vi "CRYChange Name by Calibratioin.vi"(9 "Calibration In":string, 10 "Hardware In":string, 11 "Changed Names":T2) -> ()   [LabVIEW 2013]
uses:
  CRYSystem/Typedef Control/CRYChanged Names Cluster.ctl
  CRYSystem/Typedef Control/CRYChanged Data Array Cluster.ctl
  CRYSystem/Typedef Control/CRYChanged Data Cluster.ctl
  CRYSystem/Typedef Control/CRYStimulus Type.ctl
  CRYCurveLibrary/Global/CRYCurve Library Global.vi
panel:
  in  "Ref Data Statistics":T1
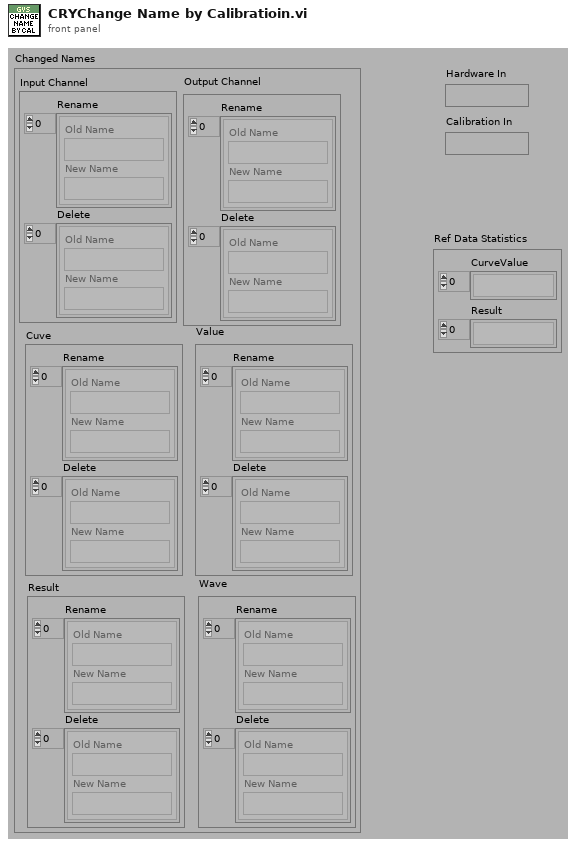
[diagram p1: front panel]
types:
  T1 = cluster{"CurveValue":string[], "Result":string[]}
  T2 = typedef "CRYChanged Names Cluster.ctl" = cluster{"Input Channel":T3, "Output Channel":T3, "Cuve":T3, "Value":T3, "Result":T3, "Wave":T3}
  T3 = typedef "CRYChanged Data Array Cluster.ctl" = cluster{"Rename":T4[], "Delete":T4[]}
  T4 = typedef "CRYChanged Data Cluster.ctl" = cluster{"Old Name":string, "New Name":string}
  T5 = typedef "CRYStep.ctl" = cluster{"No.VI":i32, "Category":string, "StepName":string, "Seq setup flattened":string, "Comment":string, "Steps config.":bool[], "Jump config":i32[], "Start":dbl, "Increment":dbl, "Name":string, "Unit":string, "Y data":u16, "Y prefix":string, "Y dB ref":dbl, "Y unit":string, "Repeat State Array":cluster{"Start":dbl, "Increment":dbl, "Count":i32, "Num":i32}[]}
  T6 = typedef "CRYStimulus Cluster.ctl" = cluster{"StimulusType":string, "UseMLValArray":u16[], "ML_axisArray":u16[], "MLValLevelNameArray":string[], "Level(U)Array":dbl[], "Start(Stop)FreqArray":dbl[], "Start(Stop)AmpArray":dbl[], "StepResolutionArray":u16[], "Unit_Array":u16[], "DegValArray":dbl[], "DegUnitArray":string[], "Steps1":i32, "Cycle/step1(#)":u32, "Time/step1(s)":dbl, "Transition1":dbl, "SweepRate2":dbl, "Freq3(Hz)":dbl, "Steps3(#)":dbl, "Cycles3(#)":u32, "StepSize3":dbl, "wave time":string, "RMS_Value4":dbl, "Peak_Value4":dbl, "WavePath4":string, "RMS_unit4":string, "Peak_unit4":string, "wave Info":string, "dc_ctrl5_1":u16, "dc_ctrl5_2":u16, "dc_polar5":u16, "Max.Current":u16, "Steps5(#)":u32, "Time/Step5":dbl, "Level5":dbl, "StepsSize5Val":dbl, "StepSize5Unit":string, "SweepType":u16, "Fixed/Ratio6":u16, "Transition6":dbl, "Steps6(#)":dbl, "Cycle/Steps6(#)":u32, "Time/Steps6(s)":dbl, "Freq6(Hz)":dbl, "Difference6(Hz)":dbl, "Ratio6":string, "NoiseType7":u16, "Duration7(s)":dbl, "MinFreq7(Hz)":dbl, "MaxFreq7(Hz)":dbl, "MinFreq8(Hz)":dbl, "MaxFreq8(Hz)":dbl, "FreqRounding8":bool, "Duration8(s)":dbl, "Tones8":dbl, "RoundingVal8":dbl, "ApplyEQ":bool, "Duration(s)":dbl, "CustomStimulusName ":string, "Flatten Element Array":string[], "sine waves":cluster{"freq":dbl, "ampl":dbl, "cycles":dbl}[], "Channel Out":i32, "RatioVal6":dbl, "TabCtrl6":enum32{"Master Tone", "Slave Tone"}, "Signal Type Name":string, "Help":string, "Channel Sel":u16, "V on DUT":bool, "Output Imp":dbl, "Nominal Imp":dbl}
  T7 = typedef "CRYfstepsw.ctl" = cluster{"Level(U)":dbl, "Start Freq(Hz)":dbl, "Stop Freq(Hz)":dbl, "ML val level name":string, "Use ML Val level?":bool, "ML axis":u8, "Steps (#)":i32, "Cycles/step(#)":u32, "Time/step (s)":dbl, "Step Resolution":u16, "unit":u16, "Start Freq Name":string, "Stop Freq Name":string, "Start Freq Axis":u8, "Stop Freq Axis":u8, "Start Freq Flag":string, "Stop Freq Flag":string, "Output Imp":dbl, "Nominal Imp":dbl, "V on DUT":bool}
  T8 = typedef "CRYflogsw.ctl" = cluster{"Level(U)":dbl, "Start Freq(Hz)":dbl, "Stop Freq(Hz)":dbl, "Sweep Rate(s/dec)":dbl, "Use ML Val level?":bool, "ML val level name":string, "ML axis":u8, "TSR params":cluster{"FSamp":dbl, "FStart":dbl, "FStop":dbl, "NOffset":dbl, "MStop":dbl, "MStart":dbl, "NHarm":dbl, "Tsamp":dbl, "Amplit":dbl}, "unit":u16, "Start Freq Name":string, "Stop Freq Name":string, "Start Freq Axis":u8, "Stop Freq Axis":u8, "Start Freq Flag":string, "Stop Freq Flag":string, "Output Imp":dbl, "Nominal Imp":dbl, "V on DUT":bool}
  T9 = typedef "CRYampsw.ctl" = cluster{"Freq(Hz)":dbl, "Steps (#)":i32, "Cycles(#)":u32, "Use ML Val freq?":bool, "ML val freq name":string, "ML axis":u8, "Start Ampl(U)":dbl, "Stop Ampl(U)":dbl, "unit":u16}
  T10 = typedef "CRYwavefile.ctl" = cluster{"Level(U)":dbl, "Wave Path":string, "ML axis":u8, "ML val level name":string, "Use ML Val level?":bool, "wave info":string, "wave time":string, "Peak value4":dbl, "RMS value4":dbl, "wave channel":u16, "unit":u16, "Output Imp":dbl, "Nominal Imp":dbl, "V on DUT":bool}
  T11 = typedef "CRYdcconn.ctl" = cluster{"dc ctrl":u16, "dcmax I":u16, "dc polar":u16, "dc ctrl":u16, "Steps (#)":i32, "Time/step (s)":dbl, "Start Ampl(U)":dbl, "Stop Ampl(U)":dbl, "Level(U)":dbl, "Step Size":dbl}
  T12 = typedef "CRYtwotone.ctl" = cluster{"Steps (#)":i32, "Tone Type":u8, "Freq2(Hz)":dbl, "Time/step (s)":dbl, "Cycles/step (#)":u32, "ML val level name":string, "Use ML Val level?":bool, "Level(U) 2":dbl, "Diff Freq(Hz)":dbl, "ML axis 2":u8, "Diff/Ratio":u8, "Level(U)":dbl, "Stop Freq(Hz)":dbl, "Ratio Val":dbl, "ML val level name 2":string, "Use ML Val level? 2":bool, "ML axis":u8, "Start Freq(Hz)":dbl, "Step Resolution":u16, "Ratio":u16, "TabCtrl6":enum32{"Master Tone", "Slave Tone"}, "unit 1":u16, "unit 2":u16, "Start Freq Name":string, "Stop Freq Name":string, "Start Freq Axis":u8, "Stop Freq Axis":u8, "Start Freq Flag":string, "Stop Freq Flag":string}
  T13 = typedef "CRYmltitone.ctl" = cluster{"Level(U)":dbl, "Min Freq(Hz)":dbl, "Max Freq(Hz)":dbl, "Duration(s)":dbl, "Freq Rounding":bool, "Rounding Val":dbl, "Profile":i32, "ML axis 2":u8, "ML val level name":string, "Use ML Val level?":bool, "ML axis":u8, "Step Resolution":u16, "unit":u16, "Start Freq Name":string, "Stop Freq Name":string, "Start Freq Axis":u8, "Stop Freq Axis":u8, "Start Freq Flag":string, "Stop Freq Flag":string, "Output Imp":dbl, "Nominal Imp":dbl, "V on DUT":bool}
  T14 = typedef "CRYnoise.ctl" = cluster{"Noise Type":u8, "Min Freq(Hz)":dbl, "Max Freq(Hz)":dbl, "Level(U)":dbl, "Duration(s)":dbl, "ML val level name":string, "Use ML Val level?":bool, "ML axis":u8, "unit":u16, "Start Freq Name":string, "Stop Freq Name":string, "Start Freq Axis":u8, "Stop Freq Axis":u8, "Start Freq Flag":string, "Stop Freq Flag":string, "Output Imp":dbl, "Nominal Imp":dbl, "V on DUT":bool}
  T15 = cluster{"fstepsw":T7, "flogsw":T8, "ampsw":T9, "wavefile":T10, "dcconn":T11, "twotone":T12, "mltitone":T13, "noise":T14, "sqwvsw":cluster{"Level(U)":dbl, "Duty Cycle":dbl, "ML val level name":string, "ML axis":u8, "Start Freq(Hz)":u32, "Stop Freq(Hz)":u32, "Use ML Val level?":bool, "Steps (#)":u32, "Cycles/step (#)":u32, "Time/step (s)":dbl, "Step Resolution":u16}, "tnbrst":cluster{"Level(U)":dbl, "ML val level name":string, "ML axis":u8, "Start Freq(Hz)":u32, "Use ML Val level?":bool, "Cycles/step (#)":u32, "Duration(s)":dbl}}
  T16 = cluster{"Data Type":string, "Version":u16, "Dimension":u8}
  T17 = typedef "CRYStimulus Type.ctl" = u16
  T18 = typedef "CRYAcquisition Cluster.ctl" = cluster{"Mode":u16, "Name":string, "use ch name":bool, "Record Time":dbl, "hide rec":bool, "hide play":bool, "rec delay":dbl, "rec pad":dbl, "dcc units":i8, "sine gen setting":string, "scope_fft setting":string, "voltmeter setting":string, "rta setting":string, "trig offset(sec)":dbl, "triggered  record":bool, "trig level":dbl, "trig unit":u8, "trig slop":bool, "trig timeout(sec)":dbl, "add record":bool, "EQ":bool, "record table":string[][], "play table":string[][], "trig channel":string, "Help":string}
  T19 = typedef "CRYAnalysis Cluster.ctl" = cluster{"Name":string, "Harmonics":dbl[], " Algorithm":u16, "delay":dbl, "THD(%)":bool, "Rub&Buzz":bool, "Imp":bool, "Imp Ref resistor":dbl, "Y data":u16, "Y prefix":string, "Y unit":string, "Y dB ref":dbl, "Custom Curve Names":string[], "har list items":string[], "Envelope":bool, "use custom unit":bool, "autodelay ch":dbl, "impulse":bool, " start ms":dbl, " stop ms":dbl, "Scaling":i32, "Default Overlap ":bool, "Advanced View":bool, "Loose Particle":bool, "Use default":bool, "Auto-Correlation(Stimulus)":bool, "Auto-Correlation(Response)":bool, "Deconvolved Response":bool, "Mic Current":bool, "M List Vaiues":u16, "Type":u16, "Delay Method":u16, "Apply Correction Out":bool, "Apply Correction In":bool, "Harmonics @ meas.frq":bool, "THD Normalized(%)":bool, "Total Distortion":bool, "THD+Noise(%)":bool, "Rub&Buzz Norm'd(%)":bool, "Standard Error":bool, "Confidence Limits":bool, "Total Diff":bool, "Total Noise":bool, "Total DFD(%)":bool, "Total IMD(%)":bool, "Total IM":bool, "Total DFD+Noise(%)":bool, "Use Channel Name":bool, "Waveform In":string, "Waveform Out":string, "Method":u16, "Spectral Scaling":u16, "Appliied Unit":u16, "Length Unit":u16, "Applied Units":u16, "Sens Item":u16, "Tab":i32, "Distance Unit":u16, "discard cycles":dbl, "Weigting":string, "Averaging Time":dbl, "Max duration":dbl, "Min duration":dbl, "Attack Threshold":dbl, "Hysteresis Up":dbl, "Fmin(Hz)":dbl, "Fmax(Hz)":dbl, "Freq.Resolution":dbl, "Over-samples Res.":dbl, "Win Resolution":dbl, "distance":dbl, "samples":dbl, "Overlap":dbl, "Record Length":dbl, "No.of FFTs":dbl, "Hz":dbl, "record delay":dbl, " Std Err":dbl, "Response":bool, "Coherent Power*":bool, "Stimulus":bool, "Measurement Confidence":bool, "Auto Spectrum(Response)*":bool, "Auto Spectrum(Stimulus)*":bool, "Cross Spectrum*":bool, "functions":bool, "Frequency Response":bool, "Non-Coherent Power*":bool, "Coherence (%)":bool, "Non-Coherence (%)":bool, "Signal-Noise Ratio (dB)":bool, "Non-Coherenct Distirtion*":bool, "Result Waveforms":bool, "Coupling":bool, "Averaging":u16, "Harmonics":i32, "Custom Curve Names":i32, "unLabel":string, "Custom Curve Names":string, "Unit":string, "Total IMD + Noise(%) ":bool, "ResponseMe":u16, "Intermod":dbl[], "Diff\n":dbl[], "Cross-Correlation":bool, "IM list items":string[], "Diff list items":string[], "TSR Window Type":string, "Help":string, "Custom Curve IDs":i32[], "Default Curve Names":string[], "Loose Particle waveform":bool, "Perceptual Rub&Buzz":bool, "Imp Auto Mode":u16, "Mic Auto Mode":u16, "Mic Ref resistor":dbl, "Curve Resolution":u16, "Curve Resolution Hz":dbl, "Polarity":bool}
  T20 = typedef "CRYWaveform Cluster.ctl" = cluster{"Waveform":cluster{"X0":dbl, "dX":dbl, "Y":sgl[]}, "X data":u16, "Y data":u16, "Y axis":u16, "X unit":string, "Y unit":string, "Y dB ref":dbl, "display Y":bool, "display X":bool, "Overload?":bool, "Test Info":string, "Step No.":i32, "Name":string, "protected":bool, "Sqc history":string[], "Signal Channel ID":i32, "Plot Settings":cluster{"Color":u32, "Interpolation":u8, "Point Style":u8, "Line Style":u8, "Point Color":u32, "Line Width":u8, "Bar Plot Style":u8, "Fill To":i16}, "AutoProtect":bool}
  T21 = typedef "CRYStimulus Test Infor Cluster.ctl" = cluster{"Stimulus Type":string, "Signal Type":string, "In/Out":bool, "FAPS":cluster{"freq":dbl, "ampl":dbl, "cycles":dbl, "samples":i32}[], "Sampling Rate":dbl, "Samples":i32, "Analysis Param":string, "Resolution":u16, "Steps":u32, "Analysis Value":dbl[], "Diff Freq":dbl, "FStart":dbl, "FStop":dbl, "Calibration Param":string, "Anti Alias":dbl, "Level Out1":dbl, "Level Out2":dbl, "EQ":bool}
  T22 = cluster{"Custom Curve Names":string, "Custom Curve IDs":i32, "Default Curve Names":string}[]
  T23 = typedef "CRYPost Processing Cluster.ctl" = cluster{"Name":string, "Op Type":u16, "Curve A":string, "Curve B":string, "Axis Mode":u16, "Work Mode":u16, "Width":u16, "Weighting win":u16, "Search Mode":u16, "Freq Mode":u16, "New Sampling Rate":dbl, "Use Default Name":bool, "x":bool, "y":bool, "z":bool, "All points":bool, "A_single val axis":u16, "B_single val axis":u16, "Use Default Value":bool, "Result Name":string, "Smoothing Width":i32, "Window":u16, "Para_dB":sgl, "Para_%":sgl, "Exponent":sgl, "Hz":dbl, "Direct Weighting":bool, "Auto Inc":bool, "Inc(deg)":i32, "Total Rotation":i32, "Ref Freq Mode":u16, "Ref Waveform":string, "Sampling Rate":dbl, "Weighting Curve":string, "Ref Freq":dbl, "Curve Group":string[], "Search Items":string[], "Custom unit info":cluster{"use custom":bool, "lin/log":u16, "unit":string, "dB ref":dbl, "common dB":u16}, "Unit":string, "Type A":enum16{"Curves", "Values", "Results", "WFM"}, "Type B":enum16{"Curves", "Values", "Results", "WFM"}, "Unary Operator":u16, "Binary Operator":u16, "Statistical Operator":u16, "Constant ":dbl, "New Resolution":u16, "user equation cluster":T24, "Help":string, "Tab Value":enum32{"Setting", "Help"}, "Zwciker_X-axis":u16, "Zwicker_spectrum":bool, "Freq Sampling Mode":u16, "Freq Sampling Rate":dbl, "Smoothing":bool, "Work in Statics":u16, "Result Data":string[]}
  T24 = typedef "CRYUser Equation Cluster.ctl" = cluster{"Custom unit input array":cluster{"use custom":bool, "lin/log":u16, "unit":string, "dB ref":dbl, "common dB":u16}[], "Custom unit results array ":cluster{"use custom":bool, "lin/log":u16, "unit":string, "dB ref":dbl, "common dB":u16}[], "Desired Result Variables":string[], "Desired Result Names":string[], "Input Curve Names":string[], "Input Curve Variables":string[], "equation":string, "Input axis":u16[], "Results axis":u16[], "# input curves":i32, "# Desired result curves ":i32, "Input Values":string[], "Result Values":string[]}
  T25 = typedef "CRYLimits.ctl" = cluster{"Name":string, "Tolerance":u16, "X Axis":u16, "Limits":u16, "Upper Limit":cluster{dbl, dbl}[], "Align Ref":cluster{dbl, dbl}, "Lower Limit":cluster{dbl, dbl}[], "Y data":u16, "Y unit":string, "Y dB ref":dbl, "Curve Names":string[], "Y-Resolution":u8, "Type":u16, "x float":bool, "X min-max-step":cluster{"Limit X Offset Min":dbl, "Limit X Offset Max":dbl, "Limit X Offset Step Size":dbl}, "magn/phase":u16, "Upper Limit Type":u16, "Lower Limit Type":u16, "Lim Curve axis up":u16, "Lim Curve axis lo":u16, "Data Selection Upper":u16, "Data Selection Lower":u16, "X-Resolution":u8, "Output failed point curves?":bool, "X data":u16, "X unit":string, "X dB ref":dbl, "X-Y Graph Set-up":string, "Tab Value":enum32{"Data", "Parameters"}, "Help":string, "X Up Val":dbl, "Y Up Val":dbl, "X Low Val":dbl, "Y Low Val":dbl, "Up Limit Val":dbl, "Low Limit Val":dbl, "bAdd DataName":bool, "Custom Name":string}
  T26 = typedef "CRYStatistic cluster.ctl" = cluster{"Mode":u16, "No.Ranked(BF)":i32, "No.Ranked(WF)":i32, "Absolute Margin Standard Deviation":bool, "+/- sigma Res":i32, "Margin Standard Deviation":bool, "Margin Mean":bool, "Overall Yield":bool, "Individual Limits Yield":bool, "LSL Unit":string, "USL Unit\n":string, "LSL":dbl, "USL":dbl, "Worst Fit to Average":bool, "Best Fit to Average":bool, "Ppk":bool, "Pp":bool, "Absolute Standard Deviation":bool, "+/- sigma Dat":i32, "Standard Deviation ":bool, "Mean":bool, "Min ":bool, "Max ":bool, "No.of Curves Selected":i32, "Curves":string[], " Results":string[], "Name":string, "Help":string, "Tab Value":enum32{"Setting", "Help"}, "Work in":u16, "Mode xyz":u16}
  T27 = typedef "CRYAuto Save Cluster.ctl" = cluster{"Name":string, "save":enum16{"Data", "Results", "Waveforms"}, "Item Names":string[], "Autosave folder":path, "data format":u16, "filename option":enum16{"auto", "prompt"}, "fn construction":i32[], "layout":enum16{"rows", "columns"}, "notation":enum16{"sci", "float"}, "precision":i32, "prompt comment":bool, "header":enum16{"none", "standard", "custom"}, "custom header":string, "serial no.":bool, "User defined":string, "delimiter":enum16{"tab", "comma", "space", "other"}, "other delim":string, "axes":cluster{"x":bool, "y":bool, "z":bool}, "Time Stamp":bool, "Lot No.":bool, "Operator":bool, "Excel Template":string, "New or Append":u16, "Data":u16, "Help":string, "Tab Value":enum32{"Setting", "Help"}, "UDL or DSN":path, "User Default":bool, "Selector":i32, "Axis":u16, "Value Name":string, "format string":cluster{"dB Format String out":string, "Lin Format String out":string}, "DBPath":path}
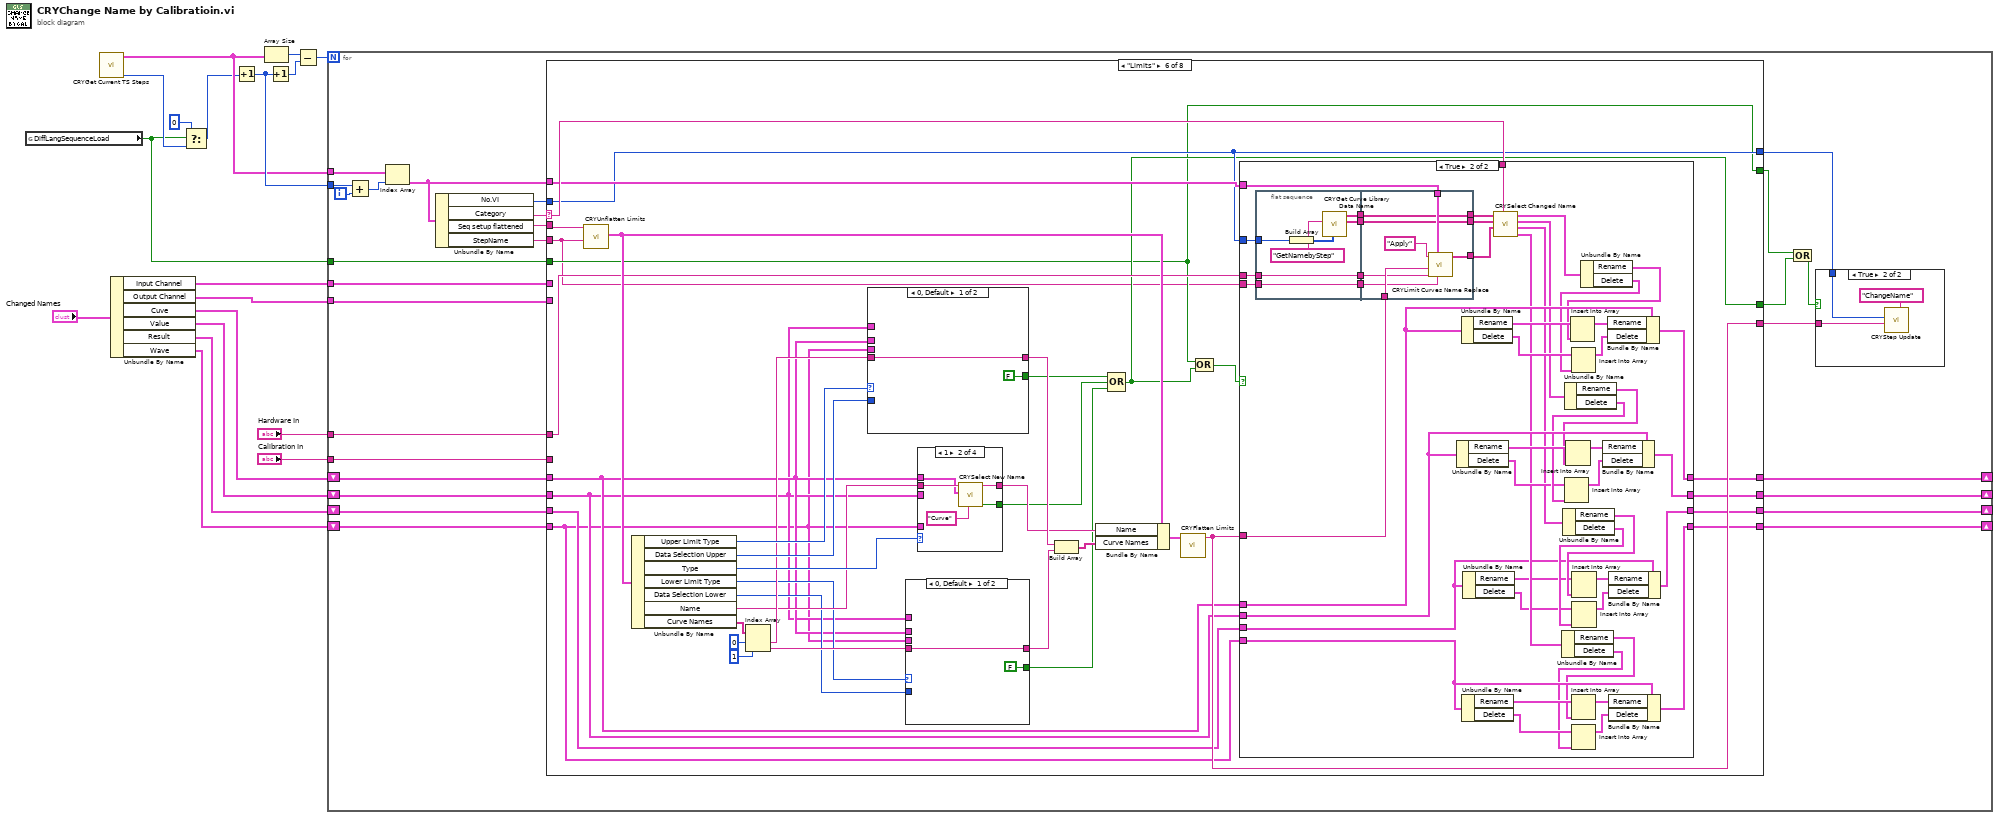
[diagram p0: block diagram]
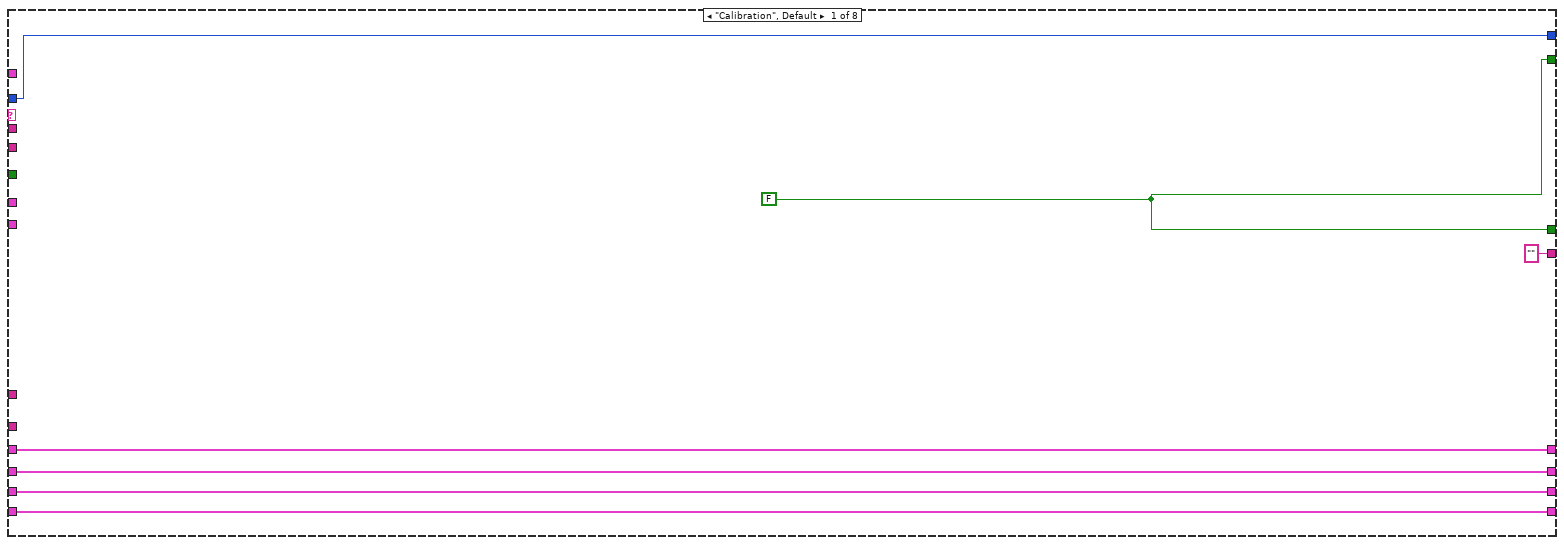
[diagram p3: hidden frame]
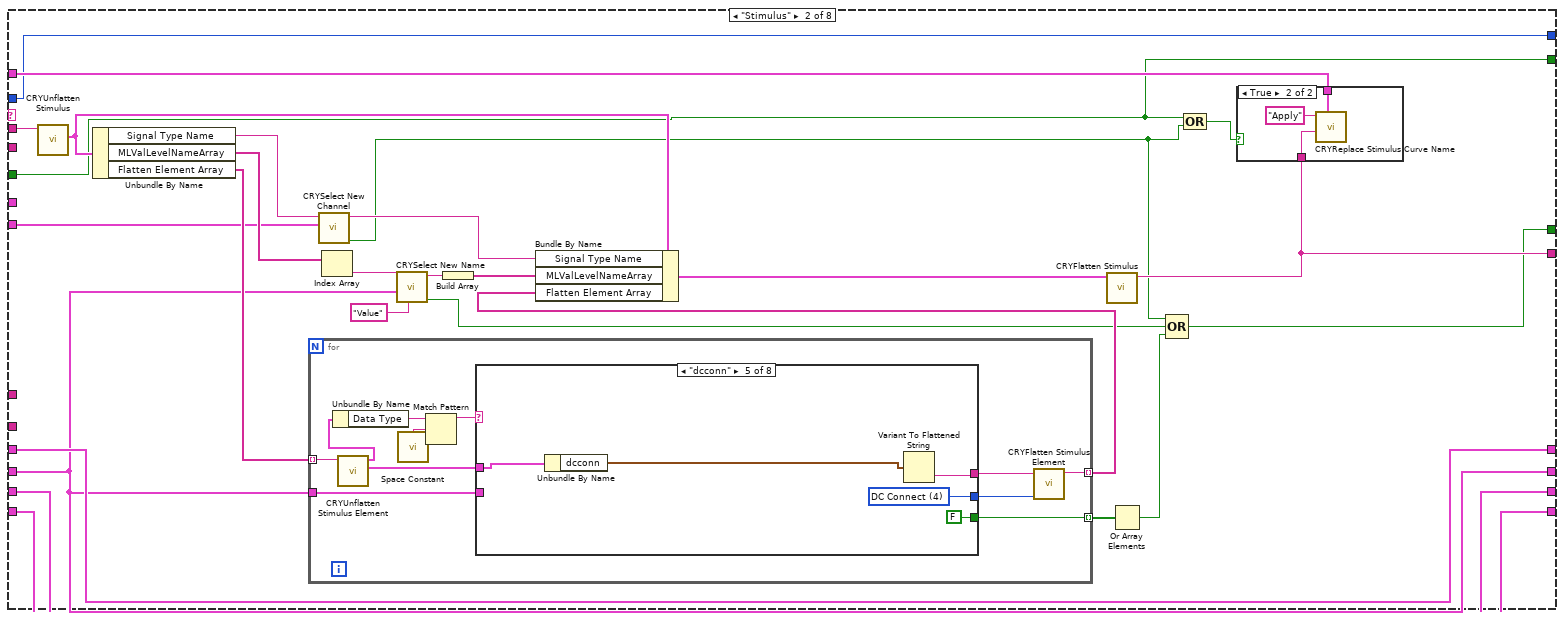
[diagram p4: hidden frame]
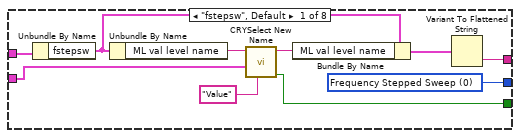
[diagram p5: hidden frame]
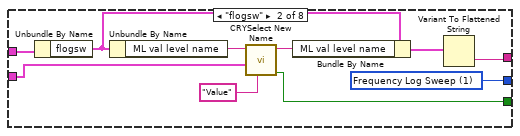
[diagram p6: hidden frame]
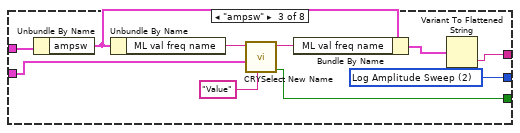
[diagram p7: hidden frame]
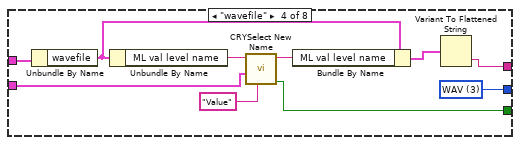
[diagram p8: hidden frame]
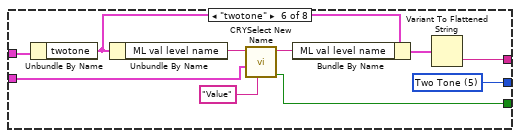
[diagram p9: hidden frame]
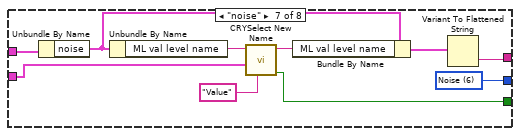
[diagram p10: hidden frame]
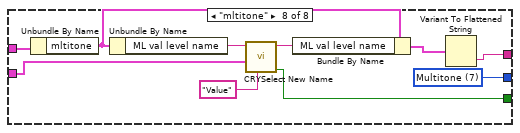
[diagram p11: hidden frame]
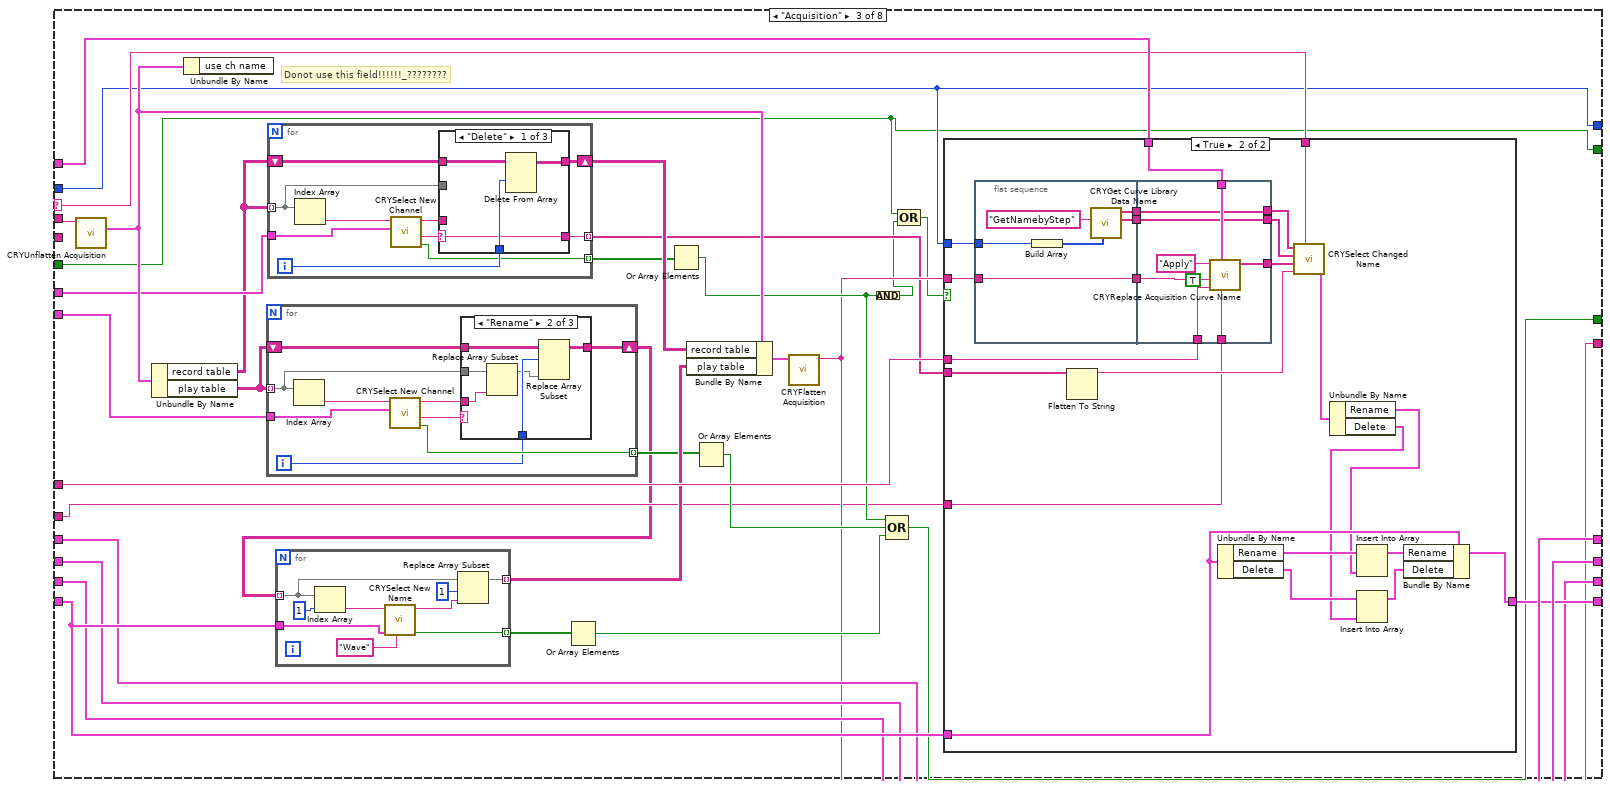
[diagram p13: hidden frame]
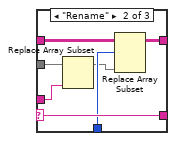
[diagram p14: hidden frame]
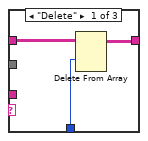
[diagram p16: hidden frame]
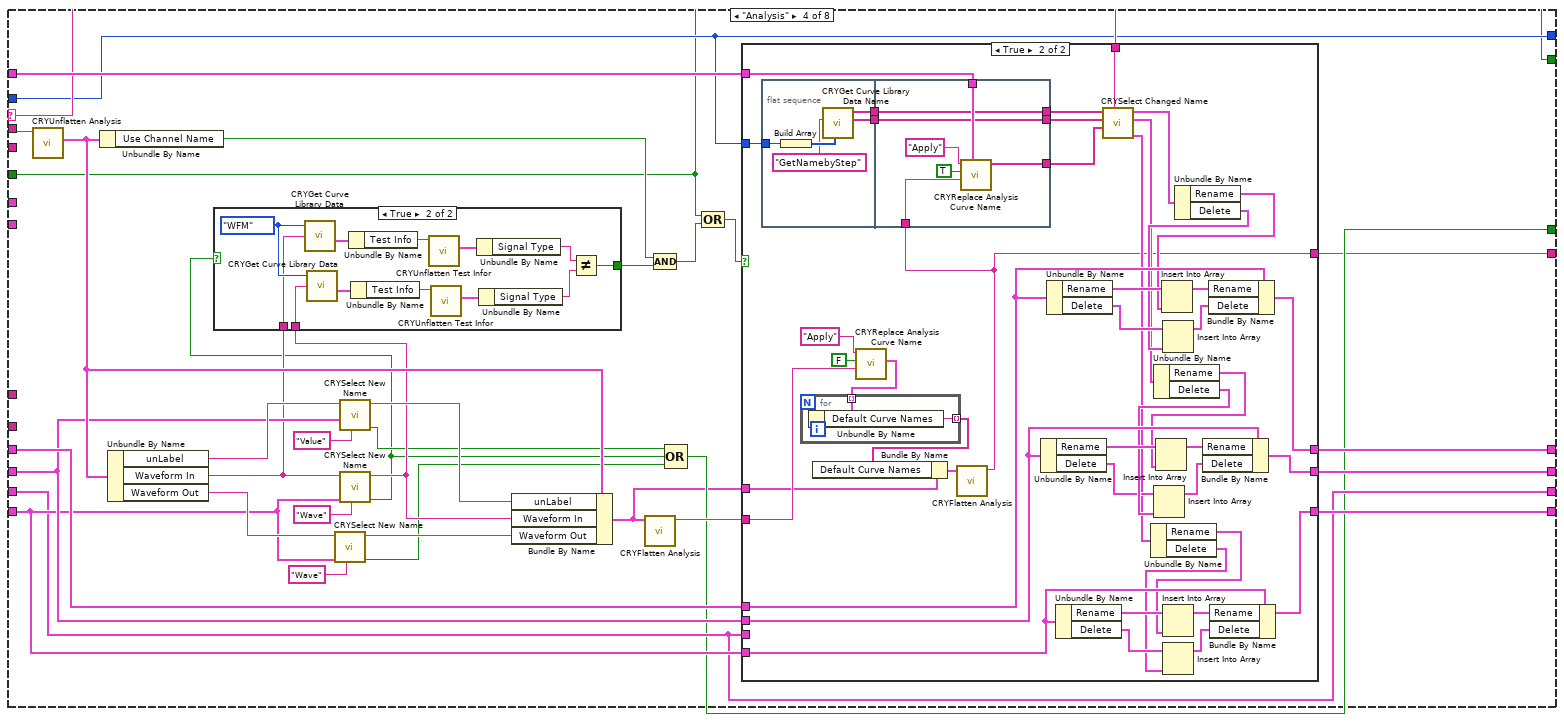
[diagram p19: hidden frame]
diagram:
  n1 = global read "CRYCurve Library Global.vi" "DiffLangSequenceLoad"() -> (w1:bool)
  n2 = call "CRYGet Current TS Steps.vi"() -> ("SelectStepNumber in Tree"=w3:i32, "Steps"=w5:T5[])  [unwired: 7 in, 3 out]
  n3 = Unbundle By Name("Changed Names") -> ("Input Channel"=w11:T3, "Output Channel"=w12:T3, "Cuve"=w14:T3, "Value"=w13:T3, "Result"=w10:T3, "Wave"=w15:T3)
  n4 = Select(t=0 ("SelectStepNumber in Tree"), s=w1, f=w3) -> (s? t:f=w2:i32)
  n5 = Increment(x=w2) -> (x+1=w6:i32)
  n6 = Array Size(array=w5) -> (size(s)=w17:i32)
  n7 = Increment(x=w6) -> (x+1=w7:i32)
  n8 = Subtract(x=w17, y=w7) -> (x-y=w16:i32)
  n9 = for {
    N: w16 -> [_]
    tunnel: "Hardware In" -> [w42]
    tunnel: w12 -> [w36]
    tunnel: w11 -> [w35]
    shift-right: [w31] -> _
    shift-left: w14 -> [w33]
    shift-right: [w30] -> _
    shift-left: w13 -> [w37]
    shift-right: [w29] -> _
    shift-left: w10 -> [w32]
    shift-right: [w28] -> _
    shift-left: w15 -> [w34]
    tunnel: "Calibration In" -> [w27]
    tunnel: w5 -> [w26]
    tunnel: w6 -> [w25]
    tunnel: w1 -> [w22]
    i -> [w40]
    n10 = Add(x=w25, y=w40) -> (x+y=w38:i32)
    n11 = Index Array(array=w26, index=w38) -> (element=w39:T5)
    n12 = Unbundle By Name(w39) -> ("No.VI"=w41:i32, "Category"=w45:string, "Seq setup flattened"=w44:string, "StepName"=w24:string)
    n13 = case shown="\"Limits\"" w45 {
      selector: w45 -> [_ _ w180 w306 w405 w554 w714 _]
      tunnel: w44 -> [_ w81 w202 w326 w444 w575 w738 w856]
      tunnel: ["" ("Auto Save flattened") w82 w182 w295 w413 w552 w724 w853] -> w43
      tunnel: w42 -> [_ _ w201 _ _ w551 _ _]
      tunnel: w41 -> [w50 w59 w175 w299 w404 w542 w712 w843]
      tunnel: [w49 w64 w183 w303 w406 w541 w711 w844] -> w21
      tunnel: w39 -> [_ w80 w200 w324 w443 w553 w737 _]
      tunnel: w37 -> [w53 w62 w191 w314 w421 w549 w727 w848]
      tunnel: w36 -> [_ w76 w199 _ _ _ _ _]
      tunnel: w35 -> [_ _ w195 _ _ _ _ _]
      tunnel: w34 -> [w51 w60 w194 w313 w420 w547 w723 w846]
      tunnel: w33 -> [w54 w63 w192 w315 w422 w550 w728 w849]
      tunnel: w32 -> [w52 w61 w189 w308 w415 w548 w713 w847]
      tunnel: [w54 w63 w192 w312 w419 w546 w726 w849] -> w31
      tunnel: [w53 w62 w191 w311 w418 w545 w725 w848] -> w30
      tunnel: [w52 w61 w189 w308 w415 w543 w713 w847] -> w29
      tunnel: [w51 w60 w190 w310 w417 w544 w723 w846] -> w28
      tunnel: w27 -> [_ _ w179 _ _ _ _ _]
      tunnel: w24 -> [_ _ _ _ _ w538 _ _]
      tunnel: [w50 w59 w175 w299 w404 w542 w712 w843] -> w23
      tunnel: w22 -> [_ w56 w172 w294 w401 w539 w709 w842]
      tunnel: [w49 w56 w172 w294 w401 w539 w709 w842] -> w19
      frame "Calibration", Default {
        w49 = FALSE
      }
      frame "Stimulus" {
        n14 = call "CRYUnflatten Stimulus.vi"("Flatten Stimulus"=w81) -> ("Stimulus"=w79:T6)  [unwired: 8 in, 2 out]
        n15 = Unbundle By Name(w79) -> ("Signal Type Name"=w75:string, "MLValLevelNameArray"=w78:string[], "Flatten Element Array"=w77:string[])
        n16 = for {
          tunnel: w77 -> [w90] mode=indexing
          tunnel: [w88] -> w71 mode=indexing
          tunnel: w62 -> [w86]
          tunnel: [w85] -> w66 mode=indexing
          n17 = call "CRYUnflatten Stimulus Element.vi"("Unflatten Stimulus Element setup"=w90) -> ("Stimulus Default"=w84:T15, "Header of common"=w93:T16)  [unwired: 1 in, 8 out]
          n18 = Unbundle By Name(w93) -> ("Data Type"=w92:string)
          n19 = call <vilib>:"Space Constant.vi"() -> ("String"=w91:string)
          n20 = Match Pattern(string=w92, regular expression=w91) -> (before substring=w89:string)  [unwired: 4 out]
          n21 = case shown="\"dcconn\"" w89 {
            tunnel: w84 -> [w102 w112 w122 w132 w136 w147 w157 w167]
            tunnel: [w101 w111 w121 w131 w138 w146 w156 w166] -> w87
            tunnel: w86 -> [w97 w107 w117 w127 _ w142 w152 w163]
            tunnel: [w96 w106 w116 w126 FALSE ("Change") w141 w151 w161] -> w85
            tunnel: [w94 w104 w114 w124 w134 w139 w149 w159] -> w83
            frame "fstepsw", Default {
              w101 = T17 0 items=["Frequency Stepped Sweep", "Frequency Log Sweep", "Log Amplitude Sweep", "WAV", "DC Connect", "Two Tone", "Noise", "Multitone"] ("Stimulus Type")
              n22 = Unbundle By Name(w102) -> ("fstepsw"=w103:T7)
              n23 = Unbundle By Name(w103) -> ("ML val level name"=w100:string)
              n24 = call "CRYSelect New Name.vi"("Type"="Value", "Value"=w97, "Name In"=w100) -> ("Change"=w96:bool, "Name Out"=w99:string)  [unwired: 6 in, 1 out]
              n25 = Bundle By Name(cluster=w103, "ML val level name"=w99) -> (w95:T7)
              n26 = Variant To Flattened String(Variant=w95) -> (data string=w94:string)  [unwired: 1 out]
            }
            frame "flogsw" {
              w111 = T17 1 items=["Frequency Stepped Sweep", "Frequency Log Sweep", "Log Amplitude Sweep", "WAV", "DC Connect", "Two Tone", "Noise", "Multitone"] ("Stimulus Type")
              n27 = Unbundle By Name(w112) -> ("flogsw"=w113:T8)
              n28 = Unbundle By Name(w113) -> ("ML val level name"=w110:string)
              n29 = call "CRYSelect New Name.vi"("Type"="Value", "Value"=w107, "Name In"=w110) -> ("Change"=w106:bool, "Name Out"=w109:string)  [unwired: 6 in, 1 out]
              n30 = Bundle By Name(cluster=w113, "ML val level name"=w109) -> (w105:T8)
              n31 = Variant To Flattened String(Variant=w105) -> (data string=w104:string)  [unwired: 1 out]
            }
            frame "ampsw" {
              w121 = T17 2 items=["Frequency Stepped Sweep", "Frequency Log Sweep", "Log Amplitude Sweep", "WAV", "DC Connect", "Two Tone", "Noise", "Multitone"] ("Stimulus Type")
              n32 = Unbundle By Name(w122) -> ("ampsw"=w123:T9)
              n33 = Unbundle By Name(w123) -> ("ML val freq name"=w120:string)
              n34 = call "CRYSelect New Name.vi"("Type"="Value", "Value"=w117, "Name In"=w120) -> ("Change"=w116:bool, "Name Out"=w119:string)  [unwired: 6 in, 1 out]
              n35 = Bundle By Name(cluster=w123, "ML val freq name"=w119) -> (w115:T9)
              n36 = Variant To Flattened String(Variant=w115) -> (data string=w114:string)  [unwired: 1 out]
            }
            frame "wavefile" {
              w131 = T17 3 items=["Frequency Stepped Sweep", "Frequency Log Sweep", "Log Amplitude Sweep", "WAV", "DC Connect", "Two Tone", "Noise", "Multitone"] ("Stimulus Type")
              n37 = Unbundle By Name(w132) -> ("wavefile"=w133:T10)
              n38 = Unbundle By Name(w133) -> ("ML val level name"=w130:string)
              n39 = call "CRYSelect New Name.vi"("Type"="Value", "Value"=w127, "Name In"=w130) -> ("Change"=w126:bool, "Name Out"=w129:string)  [unwired: 6 in, 1 out]
              n40 = Bundle By Name(cluster=w133, "ML val level name"=w129) -> (w125:T10)
              n41 = Variant To Flattened String(Variant=w125) -> (data string=w124:string)  [unwired: 1 out]
            }
            frame "dcconn" {
              w138 = T17 4 items=["Frequency Stepped Sweep", "Frequency Log Sweep", "Log Amplitude Sweep", "WAV", "DC Connect", "Two Tone", "Noise", "Multitone"] ("Stimulus Type")
              n42 = Unbundle By Name(w136) -> ("dcconn"=w135:T11)
              n43 = Variant To Flattened String(Variant=w135) -> (data string=w134:string)  [unwired: 1 out]
            }
            frame "twotone" {
              w146 = T17 5 items=["Frequency Stepped Sweep", "Frequency Log Sweep", "Log Amplitude Sweep", "WAV", "DC Connect", "Two Tone", "Noise", "Multitone"] ("Stimulus Type")
              n44 = Unbundle By Name(w147) -> ("twotone"=w148:T12)
              n45 = Unbundle By Name(w148) -> ("ML val level name"=w145:string)
              n46 = call "CRYSelect New Name.vi"("Type"="Value", "Value"=w142, "Name In"=w145) -> ("Change"=w141:bool, "Name Out"=w144:string)  [unwired: 6 in, 1 out]
              n47 = Bundle By Name(cluster=w148, "ML val level name"=w144) -> (w140:T12)
              n48 = Variant To Flattened String(Variant=w140) -> (data string=w139:string)  [unwired: 1 out]
            }
            frame "noise" {
              w156 = T17 6 items=["Frequency Stepped Sweep", "Frequency Log Sweep", "Log Amplitude Sweep", "WAV", "DC Connect", "Two Tone", "Noise", "Multitone"] ("Stimulus Type")
              n49 = Unbundle By Name(w157) -> ("noise"=w158:T14)
              n50 = Unbundle By Name(w158) -> ("ML val level name"=w155:string)
              n51 = call "CRYSelect New Name.vi"("Type"="Value", "Value"=w152, "Name In"=w155) -> ("Change"=w151:bool, "Name Out"=w154:string)  [unwired: 6 in, 1 out]
              n52 = Bundle By Name(cluster=w158, "ML val level name"=w154) -> (w150:T14)
              n53 = Variant To Flattened String(Variant=w150) -> (data string=w149:string)  [unwired: 1 out]
            }
            frame "mltitone" {
              w166 = T17 7 items=["Frequency Stepped Sweep", "Frequency Log Sweep", "Log Amplitude Sweep", "WAV", "DC Connect", "Two Tone", "Noise", "Multitone"] ("Stimulus Type")
              n54 = Unbundle By Name(w167) -> ("mltitone"=w168:T13)
              n55 = Unbundle By Name(w168) -> ("ML val level name"=w165:string)
              n56 = call "CRYSelect New Name.vi"("Type"="Value", "Value"=w163, "Name In"=w165) -> ("Change"=w161:bool, "Name Out"=w164:string)  [unwired: 6 in, 1 out]
              n57 = Bundle By Name(cluster=w168, "ML val level name"=w164) -> (w160:T13)
              n58 = Variant To Flattened String(Variant=w160) -> (data string=w159:string)  [unwired: 1 out]
            }
          }
          n59 = call "CRYFlatten Stimulus Element.vi"("Stimulus Type"=w87, "Flattened Stimulus Element"=w83) -> ("Flatten Stimulus Setup String"=w88:string)  [unwired: 9 out]
        }
        n60 = call "CRYSelect New Channel.vi"("Channel In"=w76, "Channel Name In"=w75) -> ("Change"=w58:bool, "Channel Name  Out"=w74:string)  [unwired: 7 in, 1 out]
        n61 = Index Array(array=w78) -> (element=w69:string)  [unwired: 1 in]
        n62 = call "CRYSelect New Name.vi"("Type"="Value", "Value"=w62, "Name In"=w69) -> ("Change"=w67:bool, "Name Out"=w70:string)  [unwired: 6 in, 1 out]
        n63 = Build Array(w70) -> (w72:string[])
        n64 = Bundle By Name(cluster=w79, "Signal Type Name"=w74, "MLValLevelNameArray"=w72, "Flatten Element Array"=w71) -> (w73:T6)
        n65 = call "CRYFlatten Stimulus.vi"("Stimulus"=w73) -> ("Flatten Stimulus String"=w82:string)  [unwired: 10 in]
        n66 = Or Array Elements(Boolean array=w66) -> (logical OR=w65:bool)
        n67 = Compound Arithmetic op=OR(w58, w67, w65) -> (w64:bool)
        n68 = Compound Arithmetic op=OR(w56, w58) -> (w57:bool)
        n69 = case shown="True" w57 {
          tunnel: w82 -> [_ w171]
          tunnel: w80 -> [_ w170]
          frame False {
          }
          frame True {
            n70 = call "CRYReplace Stimulus Curve Name.vi"("Setup in"=w170, "Step Setup In"=w171, "Type In"="Apply" ("Type")) -> ()  [unwired: 8 in, 1 out]
          }
        }
      }
      frame "Acquisition" {
        # "Donot use this field!!!!!!_????????"
        n71 = call "CRYUnflatten Acquisition.vi"("Flatten Acquisition"=w202) -> ("Acquisition"=w203:T18)  [unwired: 10 out]
        n72 = Unbundle By Name(w203) -> ("record table"=w178:string[][], "play table"=w177:string[][])
        n73 = Unbundle By Name(w203) -> ()  [unwired: 1 out]
        n74 = for {
          tunnel: w177 -> [w241] mode=indexing
          tunnel: w199 -> [w243]
          tunnel: [w242] -> w187 mode=indexing
          shift-right: [w239] -> w176
          shift-left: w177 -> [w240]
          i -> [w238]
          n75 = Index Array(array=w241) -> (element=w244:string)  [unwired: 1 in]
          n76 = call "CRYSelect New Channel.vi"("Channel In"=w243, "Channel Name In"=w244) -> ("Change"=w242:bool, "Status"=w236:string, "Channel Name  Out"=w237:string)  [unwired: 7 in]
          n77 = case shown="\"Rename\"" w236 {
            tunnel: w237 -> [_ w252 _]
            tunnel: w241 -> [_ w253 _]
            tunnel: w238 -> [w247 w250 _]
            tunnel: w240 -> [w246 w251 w254]
            tunnel: [w245 w249 w254] -> w239
            frame "Delete" {
              n78 = Delete From Array(array=w246, index (row)=w247) -> (array with subset deleted=w245:string[][])  [unwired: 2 in, 1 out]
            }
            frame "Rename" {
              n79 = Replace Array Subset(array=w253, new element=w252) -> (w248:string[])  [unwired: 1 in]
              n80 = Replace Array Subset(array=w251, new element=w248, index (row)=w250) -> (w249:string[][])  [unwired: 1 in]
            }
            frame "Origin", Default {
            }
          }
        }
        n81 = for {
          tunnel: w178 -> [w218] mode=indexing
          tunnel: w195 -> [w221]
          tunnel: [w216] -> w193 mode=indexing
          tunnel: [w215] -> w181 mode=indexing
          shift-right: [w213] -> w197
          shift-left: w178 -> [w214]
          i -> [w217]
          n82 = Index Array(array=w218) -> (element=w222:string)  [unwired: 1 in]
          n83 = call "CRYSelect New Channel.vi"("Channel In"=w221, "Channel Name In"=w222) -> ("Change"=w216:bool, "Status"=w220:string, "Channel Name  Out"=w219:string)  [unwired: 7 in]
          n84 = case shown="\"Delete\"" w220 {
            selector: w220 -> [w225 w231 w235]
            tunnel: w219 -> [_ w232 _]
            tunnel: w218 -> [_ w233 _]
            tunnel: w217 -> [w226 w229 _]
            tunnel: [w225 w231 w235] -> w215
            tunnel: w214 -> [w224 w230 w234]
            tunnel: [w223 w228 w234] -> w213
            frame "Delete" {
              n85 = Delete From Array(array=w224, index (row)=w226) -> (array with subset deleted=w223:string[][])  [unwired: 2 in, 1 out]
            }
            frame "Rename" {
              n86 = Replace Array Subset(array=w233, new element=w232) -> (w227:string[])  [unwired: 1 in]
              n87 = Replace Array Subset(array=w230, new element=w227, index (row)=w229) -> (w228:string[][])  [unwired: 1 in]
            }
            frame "Origin", Default {
            }
          }
        }
        n88 = for {
          tunnel: w176 -> [w209] mode=indexing
          tunnel: w194 -> [w205]
          tunnel: [w207] -> w196 mode=indexing
          tunnel: [w204] -> w188 mode=indexing
          n89 = Index Array(array=w209, index=1) -> (element=w211:string)
          n90 = call "CRYSelect New Name.vi"("Type"="Wave", "Wave"=w205, "Name In"=w211) -> ("Change"=w204:bool, "Name Out"=w208:string)  [unwired: 6 in, 1 out]
          n91 = Replace Array Subset(array=w209, new element=w208, index=1) -> (w207:string[])
        }
        n92 = Or Array Elements(Boolean array=w188) -> (logical OR=w186:bool)
        n93 = Or Array Elements(Boolean array=w193) -> (logical OR=w184:bool)
        n94 = Bundle By Name(cluster=w203, "record table"=w197, "play table"=w196) -> (w198:T18)
        n95 = Or Array Elements(Boolean array=w187) -> (logical OR=w185:bool)
        n96 = call "CRYFlatten Acquisition.vi"("Acquisition"=w198) -> ("Acquisition flattened"=w182:string)  [unwired: 10 out]
        n97 = Compound Arithmetic op=AND(w184) -> (w174:bool)
        n98 = Compound Arithmetic op=OR(w184, w185, w186) -> (w183:bool)
        n99 = Compound Arithmetic op=OR(w172, w174) -> (w173:bool)
        n100 = case shown="True" w173 {
          tunnel: w182 -> [_ w276]
          tunnel: w175 -> [_ w275]
          tunnel: w201 -> [_ w274]
          tunnel: w200 -> [_ w273]
          tunnel: w194 -> [w255 w270]
          tunnel: [w255 w268] -> w190
          tunnel: w181 -> [_ w258]
          tunnel: w180 -> [_ w259]
          tunnel: w179 -> [_ w256]
          frame False {
          }
          frame True {
            n101 = flat-sequence {
              tunnel: w276 -> [w284]
              tunnel: [w283] -> w278
              tunnel: [w284] -> w277
              tunnel: w275 -> [w282]
              tunnel: [w280] -> w269
              tunnel: w274 -> [w292]
              tunnel: w278 -> [w288]
              tunnel: w277 -> [w291]
              tunnel: w273 -> [w290]
              tunnel: w269 -> [w289]
              tunnel: [w289] -> w267
              tunnel: [w288] -> w266
              tunnel: [w287] -> w265
              tunnel: w256 -> [w286]
              frame #0 {
                n102 = Build Array(w282) -> (w281:i32[])
                n103 = call "CRYGet Curve Library Data Name.vi"("nData"=w281, "sAction"="GetNamebyStep" ("sOption")) -> ("sNames"=w283:string[], "Type Out"=w280:string[])  [unwired: 6 in, 2 out]
              }
              frame #1 {
                n104 = call "CRYReplace Acquisition Curve Name.vi"("Calibration in"=w286, "Setup in"=w290, "Hardware Setup In"=w292, "Step Setup In"=w291, "No Insert CurveLib?"=TRUE, "Type In"="Apply") -> ("Inserted Names Out"=w287:string[])  [unwired: 3 in, 2 out]
              }
            }
            n105 = Flatten To String(anything=w258) -> (data string=w257:string)  [unwired: 3 in, 2 out]
            n106 = Unbundle By Name(w270) -> ("Rename"=w272:T4[], "Delete"=w264:T4[])
            n107 = call "CRYSelect Changed Name.vi"("Option"=w259, "Ref Data"=w257, "Inserted Name"=w265, "Origin Name"=w266, "Type"=w267) -> ("Wave"=w262:T3)  [unwired: 3 in, 3 out]
            n108 = Unbundle By Name(w262) -> ("Rename"=w261:T4[], "Delete"=w260:T4[])
            n109 = Insert Into Array(array=w272, new element=w261) -> (w271:T4[])  [unwired: 1 in]
            n110 = Insert Into Array(array=w264, new element=w260) -> (w263:T4[])  [unwired: 1 in]
            n111 = Bundle By Name(cluster=w270, "Rename"=w271, "Delete"=w263) -> (w268:T3)
          }
        }
      }
      frame "Analysis" {
        n112 = call "CRYUnflatten Analysis.vi"("Unflatten Analysis"=w326) -> ("Analysis"=w319:T19)  [unwired: 8 in, 2 out]
        n113 = Unbundle By Name(w319) -> ("Use Channel Name"=w325:bool)
        n114 = Unbundle By Name(w319) -> ("unLabel"=w323:string, "Waveform In"=w304:string, "Waveform Out"=w322:string)
        n115 = call "CRYSelect New Name.vi"("Type"="Wave", "Wave"=w313, "Name In"=w322) -> ("Change"=w300:bool, "Name Out"=w321:string)  [unwired: 6 in, 1 out]
        n116 = call "CRYSelect New Name.vi"("Type"="Value", "Value"=w314, "Name In"=w323) -> ("Change"=w302:bool, "Name Out"=w320:string)  [unwired: 6 in, 1 out]
        n117 = call "CRYSelect New Name.vi"("Type"="Wave", "Wave"=w313, "Name In"=w304) -> ("Change"=w301:bool, "Name Out"=w307:string)  [unwired: 6 in, 1 out]
        n118 = case shown="True" w301 {
          selector: w301 -> [w327 _]
          tunnel: w307 -> [_ w329]
          tunnel: [w327 w330] -> w305
          tunnel: w304 -> [_ w328]
          frame False {
          }
          frame True {
            w333 = enum16{"Curves", "Values", "Results", "WFM"}."WFM" ("Type")
            n119 = call "CRYGet Curve Library Data.vi"("Type"=w333, "Data Name"=w328) -> ("Wave"=w339:T20)  [unwired: 4 out]
            n120 = call "CRYGet Curve Library Data.vi"("Type"=w333, "Data Name"=w329) -> ("Wave"=w334:T20)  [unwired: 4 out]
            n121 = Unbundle By Name(w339) -> ("Test Info"=w338:string)
            n122 = Unbundle By Name(w334) -> ("Test Info"=w335:string)
            n123 = call "CRYUnflatten Test Infor.vi"("Falattend test infor"=w338) -> ("unflattened test infor data"=w337:T21)  [unwired: 9 out]
            n124 = call "CRYUnflatten Test Infor.vi"("Falattend test infor"=w335) -> ("unflattened test infor data"=w336:T21)  [unwired: 9 out]
            n125 = Unbundle By Name(w337) -> ("Signal Type"=w332:string)
            n126 = Unbundle By Name(w336) -> ("Signal Type"=w331:string)
            n127 = Not Equal?(x=w332, y=w331) -> (x != y?=w330:bool)
          }
        }
        n128 = Bundle By Name(cluster=w319, "unLabel"=w320, "Waveform In"=w307, "Waveform Out"=w321) -> (w296:T19)
        n129 = call "CRYFlatten Analysis.vi"("Analysis"=w296) -> ("Analysis flattened"=w309:string)  [unwired: 10 in]
        n130 = Compound Arithmetic op=AND(w325, w305) -> (w298:bool)
        n131 = Compound Arithmetic op=OR(w302, w301, w300) -> (w303:bool)
        n132 = Compound Arithmetic op=OR(w294, w298) -> (w297:bool)
        n133 = case shown="True" w297 {
          tunnel: w299 -> [_ w385]
          tunnel: w324 -> [_ w384]
          tunnel: w315 -> [w343 w379]
          tunnel: w314 -> [w342 w370]
          tunnel: w308 -> [_ _]
          tunnel: w313 -> [w341 w369]
          tunnel: [w343 w377] -> w312
          tunnel: [w342 w372] -> w311
          tunnel: [w341 w371] -> w310
          tunnel: w309 -> [w340 w348]
          tunnel: w306 -> [_ w354]
          tunnel: w296 -> [_ w346]
          tunnel: [w340 w344] -> w295
          frame False {
          }
          frame True {
            n134 = flat-sequence {
              tunnel: [w391] -> w386
              tunnel: w385 -> [w393]
              tunnel: [w390] -> w383
              tunnel: w386 -> [w395]
              tunnel: w344 -> [w400]
              tunnel: w384 -> [w398]
              tunnel: w383 -> [w396]
              tunnel: [w396] -> w382
              tunnel: [w395] -> w381
              tunnel: [w394] -> w353
              frame #0 {
                n135 = Build Array(w393) -> (w392:i32[])
                n136 = call "CRYGet Curve Library Data Name.vi"("nData"=w392, "sAction"="GetNamebyStep" ("sOption")) -> ("sNames"=w391:string[], "Type Out"=w390:string[])  [unwired: 6 in, 2 out]
              }
              frame #1 {
                n137 = call "CRYReplace Analysis Curve Name.vi"("Setup in"=w398, "Step Setup In"=w400, "InsertSocket?"=TRUE, "Type In"="Apply") -> ("Inserted Names Out"=w394:string[])  [unwired: 3 in, 4 out]
              }
            }
            n138 = call "CRYReplace Analysis Curve Name.vi"("Step Setup In"=w348, "InsertSocket?"=FALSE, "Type In"="Apply") -> ("Curve Info Array Out"=w351:T22)  [unwired: 4 in, 4 out]
            n139 = for {
              tunnel: w351 -> [w388] mode=indexing
              tunnel: [w387] -> w347 mode=indexing
              n140 = Unbundle By Name(w388) -> ("Default Curve Names"=w387:string)
            }
            n141 = Bundle By Name(cluster=w346, "Default Curve Names"=w347) -> (w345:T19)
            n142 = call "CRYFlatten Analysis.vi"("Analysis"=w345) -> ("Analysis flattened"=w344:string)  [unwired: 10 in]
            n143 = Unbundle By Name(w370) -> ("Rename"=w375:T4[], "Delete"=w361:T4[])
            n144 = Unbundle By Name(w379) -> ("Rename"=w380:T4[], "Delete"=w367:T4[])
            n145 = Unbundle By Name(w369) -> ("Rename"=w373:T4[], "Delete"=w358:T4[])
            n146 = call "CRYSelect Changed Name.vi"("Option"=w354, "Inserted Name"=w353, "Origin Name"=w381, "Type"=w382) -> ("Wave"=w359:T3, "Value"=w364:T3, "Cuve"=w352:T3)  [unwired: 4 in, 1 out]
            n147 = Unbundle By Name(w359) -> ("Rename"=w356:T4[], "Delete"=w355:T4[])
            n148 = Unbundle By Name(w364) -> ("Rename"=w363:T4[], "Delete"=w362:T4[])
            n149 = Insert Into Array(array=w361, new element=w362) -> (w360:T4[])  [unwired: 1 in]
            n150 = Insert Into Array(array=w375, new element=w363) -> (w376:T4[])  [unwired: 1 in]
            n151 = Insert Into Array(array=w373, new element=w356) -> (w374:T4[])  [unwired: 1 in]
            n152 = Insert Into Array(array=w358, new element=w355) -> (w357:T4[])  [unwired: 1 in]
            n153 = Unbundle By Name(w352) -> ("Rename"=w368:T4[], "Delete"=w366:T4[])
            n154 = Insert Into Array(array=w380, new element=w368) -> (w378:T4[])  [unwired: 1 in]
            n155 = Insert Into Array(array=w367, new element=w366) -> (w365:T4[])  [unwired: 1 in]
            n156 = Bundle By Name(cluster=w370, "Rename"=w376, "Delete"=w360) -> (w372:T3)
            n157 = Bundle By Name(cluster=w379, "Rename"=w378, "Delete"=w365) -> (w377:T3)
            n158 = Bundle By Name(cluster=w369, "Rename"=w374, "Delete"=w357) -> (w371:T3)
          }
        }
      }
      frame "Post Processing" {
        w433 = "_" ("string")
        w425 = "Post Processing" ("Type")
        n159 = call "CRYUnflatten Post Processing.vi"("Unflatten Post Processing"=w444) -> ("Post-Processing"=w437:T23)  [unwired: 8 in, 2 out]
        n160 = Unbundle By Name(w437) -> ("Op Type"=w424:u16, "Curve A"=w442:string, "Curve B"=w441:string, "Weighting Curve"=w440:string, "Curve Group"=w429:string[], "Ref Waveform"=w436:string, "Use Default Name"=w423:bool)
        n161 = Number To Decimal String(number=w424) -> (decimal integer string=w427:string)  [unwired: 1 in]
        n162 = Concatenate Strings(w427, w433, "B" ("string")) -> (w430:string)
        n163 = case shown="0, 1, 5, 12" w424 {
          tunnel: w441 -> [w475 w477]
          tunnel: [w474 w477] -> w439
          tunnel: w425 -> [w473 _]
          tunnel: w430 -> [w472 _]
          tunnel: w421 -> [w471 _]
          tunnel: w422 -> [w470 _]
          tunnel: w420 -> [w469 _]
          tunnel: [w468 FALSE ("Change")] -> w411
          frame 0, 1, 5, 12 {
            n164 = call "CRYSelect New Name.vi"("Type"=w473, "Option"=w472, "Wave"=w469, "Value"=w471, "Curve"=w470, "Name In"=w475) -> ("Change"=w468:bool, "Name Out"=w474:string)  [unwired: 3 in, 1 out]
          }
          frame Default {
          }
        }
        n165 = Concatenate Strings(w427, w433, "A" ("string")) -> (w431:string)
        n166 = case shown="Default" w424 {
          tunnel: w442 -> [w485 w487]
          tunnel: w425 -> [w484 _]
          tunnel: w431 -> [w483 _]
          tunnel: w421 -> [w482 _]
          tunnel: w422 -> [w481 _]
          tunnel: w420 -> [w480 _]
          tunnel: [w479 w487] -> w426
          tunnel: [w478 FALSE ("Change")] -> w412
          frame Default {
            n167 = call "CRYSelect New Name.vi"("Type"=w484, "Option"=w483, "Wave"=w480, "Value"=w482, "Curve"=w481, "Name In"=w485) -> ("Change"=w478:bool, "Name Out"=w479:string)  [unwired: 3 in, 1 out]
          }
          frame 6 {
          }
        }
        n168 = case shown="Default" w424 {
          tunnel: w436 -> [w450 w451]
          tunnel: [w449 w451] -> w435
          tunnel: w427 -> [w448 _]
          tunnel: w420 -> [w447 _]
          tunnel: w425 -> [w446 _]
          tunnel: [w445 _] -> w410
          frame 12 {
            n169 = call "CRYSelect New Name.vi"("Type"=w446, "Option"=w448, "Wave"=w447, "Name In"=w450) -> ("Change"=w445:bool, "Name Out"=w449:string)  [unwired: 5 in, 1 out]
          }
          frame Default {
          }
        }
        n170 = case shown="9" w424 {
          tunnel: w440 -> [w453 w462]
          tunnel: [w453 w461] -> w438
          tunnel: w429 -> [w452 w460]
          tunnel: [w452 w459] -> w428
          tunnel: w427 -> [_ w458]
          tunnel: w422 -> [_ w457]
          tunnel: w425 -> [_ w456]
          tunnel: [_ w455] -> w408
          tunnel: [_ w454] -> w409
          frame Default {
          }
          frame 9 {
            n171 = for {
              tunnel: w460 -> [w467] mode=indexing
              tunnel: [w466] -> w459 mode=indexing
              tunnel: w458 -> [w465]
              tunnel: w457 -> [w464]
              tunnel: [w463] -> w454 mode=indexing
              n172 = call "CRYSelect New Name.vi"("Option"=w465, "Curve"=w464, "Name In"=w467) -> ("Change"=w463:bool, "Name Out"=w466:string)  [unwired: 6 in, 1 out]
            }
            n173 = call "CRYSelect New Name.vi"("Type"=w456, "Option"=w458, "Curve"=w457, "Name In"=w462) -> ("Change"=w455:bool, "Name Out"=w461:string)  [unwired: 5 in, 1 out]
          }
        }
        n174 = Or Array Elements(Boolean array=w409) -> (logical OR=w407:bool)
        n175 = Compound Arithmetic op=OR(w412, w411, w408, w407, w410) -> (w406:bool)
        n176 = Bundle By Name(cluster=w437, "Curve A"=w426, "Curve B"=w439, "Weighting Curve"=w438, "Curve Group"=w428, "Ref Waveform"=w435) -> (w414:T23)
        n177 = Or(x=w412, y=w411) -> (x .or. y?=w416:bool)
        n178 = call "CRYFlatten Post Processing.vi"("Post-Processing"=w414) -> ("Post Processing flattened"=w413:string)  [unwired: 10 in]
        n179 = Compound Arithmetic op=AND(w416, w423) -> (w403:bool)
        n180 = Compound Arithmetic op=OR(w401, w403) -> (w402:bool)
        n181 = case shown="True" w402 {
          tunnel: w404 -> [_ w526]
          tunnel: w443 -> [_ w525]
          tunnel: w422 -> [w490 w518]
          tunnel: w421 -> [w489 w517]
          tunnel: w420 -> [w488 w516]
          tunnel: [w490 w515] -> w419
          tunnel: [w489 w514] -> w418
          tunnel: [w488 w513] -> w417
          tunnel: w413 -> [_ w491]
          tunnel: w405 -> [_ w492]
          frame False {
          }
          frame True {
            n182 = flat-sequence {
              tunnel: w526 -> [w531]
              tunnel: [w529] -> w512
              tunnel: [w528] -> w511
              tunnel: w491 -> [w537]
              tunnel: w525 -> [w535]
              tunnel: w512 -> [w534]
              tunnel: w511 -> [w533]
              tunnel: [w534] -> w510
              tunnel: [w533] -> w509
              tunnel: [w532] -> w508
              frame #0 {
                n183 = Build Array(w531) -> (w530:i32[])
                n184 = call "CRYGet Curve Library Data Name.vi"("nData"=w530, "sAction"="GetNamebyStep" ("sOption")) -> ("sNames"=w528:string[], "Type Out"=w529:string[])  [unwired: 6 in, 2 out]
              }
              frame #1 {
                n185 = call "CRYPost Processing Curve Name Replace.vi"("Setup in"=w535, "Step Setup in"=w537, "Type In"="Apply") -> ("Inserted Names Out"=w532:string[])  [unwired: 8 in]
              }
            }
            n186 = Unbundle By Name(w517) -> ("Rename"=w522:T4[], "Delete"=w500:T4[])
            n187 = Unbundle By Name(w518) -> ("Rename"=w519:T4[], "Delete"=w505:T4[])
            n188 = Unbundle By Name(w516) -> ("Rename"=w524:T4[], "Delete"=w494:T4[])
            n189 = call "CRYSelect Changed Name.vi"("Option"=w492, "Inserted Name"=w508, "Origin Name"=w509, "Type"=w510) -> ("Wave"=w497:T3, "Value"=w502:T3, "Cuve"=w507:T3)  [unwired: 4 in, 1 out]
            n190 = Unbundle By Name(w497) -> ("Rename"=w496:T4[], "Delete"=w495:T4[])
            n191 = Unbundle By Name(w502) -> ("Rename"=w501:T4[], "Delete"=w499:T4[])
            n192 = Insert Into Array(array=w522, new element=w501) -> (w521:T4[])  [unwired: 1 in]
            n193 = Insert Into Array(array=w500, new element=w499) -> (w498:T4[])  [unwired: 1 in]
            n194 = Insert Into Array(array=w524, new element=w496) -> (w523:T4[])  [unwired: 1 in]
            n195 = Insert Into Array(array=w494, new element=w495) -> (w493:T4[])  [unwired: 1 in]
            n196 = Unbundle By Name(w507) -> ("Rename"=w506:T4[], "Delete"=w503:T4[])
            n197 = Insert Into Array(array=w519, new element=w506) -> (w520:T4[])  [unwired: 1 in]
            n198 = Insert Into Array(array=w505, new element=w503) -> (w504:T4[])  [unwired: 1 in]
            n199 = Bundle By Name(cluster=w517, "Rename"=w521, "Delete"=w498) -> (w514:T3)
            n200 = Bundle By Name(cluster=w518, "Rename"=w520, "Delete"=w504) -> (w515:T3)
            n201 = Bundle By Name(cluster=w516, "Rename"=w523, "Delete"=w493) -> (w513:T3)
          }
        }
      }
      frame "Limits" {
        n202 = call "CRYUnflatten Limits.vi"("Step Name"=w538, "Unflatten Limits"=w575) -> ("Limits"=w573:T25)  [unwired: 7 in, 2 out]
        n203 = Unbundle By Name(w573) -> ("Upper Limit Type"=w571:u16, "Data Selection Upper"=w570:u16, "Type"=w572:u16, "Lower Limit Type"=w559:u16, "Data Selection Lower"=w558:u16, "Name"=w563:string, "Curve Names"=w569:string[])
        n204 = Index Array(array=w569, index #1=0 ("index"), index #2=1 ("index")) -> (element #1=w566:string, element #2=w561:string)
        n205 = case shown="0, Default" w571 {
          tunnel: w570 -> [_ w676]
          tunnel: w549 -> [_ w675]
          tunnel: w566 -> [w669 w674]
          tunnel: [w669 w673] -> w565
          tunnel: w550 -> [_ w672]
          tunnel: w547 -> [_ w671]
          tunnel: [FALSE ("Change") w670] -> w557
          frame 0, Default {
          }
          frame 1 {
            n206 = case shown="1" w676 {
              tunnel: w675 -> [w680 _ _]
              tunnel: w674 -> [w679 w685 w690]
              tunnel: [w678 w684 w689] -> w673
              tunnel: w672 -> [_ w683 _]
              tunnel: w671 -> [_ _ w688]
              tunnel: [w677 w682 w687] -> w670
              frame 0, Default {
                n207 = call "CRYSelect New Name.vi"("Type"="Value", "Value"=w680, "Name In"=w679) -> ("Change"=w677:bool, "Name Out"=w678:string)  [unwired: 6 in, 1 out]
              }
              frame 1 {
                n208 = call "CRYSelect New Name.vi"("Type"="Curve", "Curve"=w683, "Name In"=w685) -> ("Change"=w682:bool, "Name Out"=w684:string)  [unwired: 6 in, 1 out]
              }
              frame 2 {
                n209 = call "CRYSelect New Name.vi"("Type"="Wave", "Wave"=w688, "Name In"=w690) -> ("Change"=w687:bool, "Name Out"=w689:string)  [unwired: 6 in, 1 out]
              }
            }
          }
        }
        n210 = case shown="0, Default" w559 {
          tunnel: w558 -> [_ w652]
          tunnel: w549 -> [_ w651]
          tunnel: w561 -> [w645 w650]
          tunnel: [w645 w649] -> w560
          tunnel: w550 -> [_ w648]
          tunnel: w547 -> [_ w647]
          tunnel: [FALSE ("Change") w646] -> w555
          frame 0, Default {
          }
          frame 1 {
            n211 = case shown="2" w652 {
              tunnel: w651 -> [w656 _ _]
              tunnel: w650 -> [w655 w661 w666]
              tunnel: [w654 w660 w665] -> w649
              tunnel: w648 -> [_ w659 _]
              tunnel: w647 -> [_ _ w664]
              tunnel: [w653 w658 w663] -> w646
              frame 0, Default {
                n212 = call "CRYSelect New Name.vi"("Type"="Value", "Value"=w656, "Name In"=w655) -> ("Change"=w653:bool, "Name Out"=w654:string)  [unwired: 6 in, 1 out]
              }
              frame 1 {
                n213 = call "CRYSelect New Name.vi"("Type"="Curve", "Curve"=w659, "Name In"=w661) -> ("Change"=w658:bool, "Name Out"=w660:string)  [unwired: 6 in, 1 out]
              }
              frame 2 {
                n214 = call "CRYSelect New Name.vi"("Type"="Wave", "Wave"=w664, "Name In"=w666) -> ("Change"=w663:bool, "Name Out"=w665:string)  [unwired: 6 in, 1 out]
              }
            }
          }
        }
        n215 = case shown="1" w572 {
          tunnel: w550 -> [_ w697 _ _]
          tunnel: w549 -> [w693 _ _ _]
          tunnel: w547 -> [_ _ w703 _]
          tunnel: w563 -> [w695 w700 w705 w708]
          tunnel: [w694 w699 w704 w708] -> w562
          tunnel: [w692 w698 w702 FALSE ("Change")] -> w556
          frame 0 {
            n216 = call "CRYSelect New Name.vi"("Type"="Value", "Value"=w693, "Name In"=w695) -> ("Change"=w692:bool, "Name Out"=w694:string)  [unwired: 6 in, 1 out]
          }
          frame 1 {
            n217 = call "CRYSelect New Name.vi"("Type"="Curve", "Curve"=w697, "Name In"=w700) -> ("Change"=w698:bool, "Name Out"=w699:string)  [unwired: 6 in, 1 out]
          }
          frame 2 {
            n218 = call "CRYSelect New Name.vi"("Type"="Wave", "Wave"=w703, "Name In"=w705) -> ("Change"=w702:bool, "Name Out"=w704:string)  [unwired: 6 in, 1 out]
          }
          frame Default {
          }
        }
        n219 = Build Array(w565, w560) -> (w564:string[])
        n220 = Bundle By Name(cluster=w573, "Name"=w562, "Curve Names"=w564) -> (w574:T25)
        n221 = Compound Arithmetic op=OR(w557, w556, w555) -> (w541:bool)
        n222 = call "CRYFlatten Limits.vi"("Limits"=w574) -> ("Flatten Limits String"=w552:string)  [unwired: 10 in]
        n223 = Compound Arithmetic op=OR(w539, w541) -> (w540:bool)
        n224 = case shown="True" w540 {
          tunnel: w542 -> [_ w627]
          tunnel: w553 -> [_ w626]
          tunnel: w550 -> [w579 w620]
          tunnel: w549 -> [w578 w611]
          tunnel: w547 -> [w577 w610]
          tunnel: [w579 w618] -> w546
          tunnel: [w578 w613] -> w545
          tunnel: [w577 w612] -> w544
          tunnel: w552 -> [_ w609]
          tunnel: w554 -> [_ w593]
          tunnel: w551 -> [_ w591]
          tunnel: w548 -> [w576 w584]
          tunnel: [w576 w582] -> w543
          tunnel: w538 -> [_ w581]
          frame False {
          }
          frame True {
            n225 = flat-sequence {
              tunnel: [w633] -> w628
              tunnel: w627 -> [w635]
              tunnel: [w632] -> w625
              tunnel: [w630] -> w592
              tunnel: w591 -> [w630]
              tunnel: w581 -> [w629]
              tunnel: [w629] -> w580
              tunnel: w628 -> [w640]
              tunnel: w609 -> [w638]
              tunnel: w626 -> [w642]
              tunnel: w625 -> [w641]
              tunnel: [w641] -> w624
              tunnel: [w640] -> w623
              tunnel: [w639] -> w622
              tunnel: w592 -> [w637]
              tunnel: w580 -> [w636]
              frame #0 {
                n226 = Build Array(w635) -> (w634:i32[])
                n227 = call "CRYGet Curve Library Data Name.vi"("nData"=w634, "sAction"="GetNamebyStep" ("sOption")) -> ("sNames"=w633:string[], "Type Out"=w632:string[])  [unwired: 6 in, 2 out]
              }
              frame #1 {
                n228 = call "CRYLimit Curves Name Replace.vi"("StepName"=w636, "Setup in"=w642, "Hardware Setup In"=w637, "Step Set up In"=w638, "Type In"="Apply") -> ("Inserted Names Out"=w639:string[])  [unwired: 6 in]
              }
            }
            n229 = Unbundle By Name(w611) -> ("Rename"=w616:T4[], "Delete"=w600:T4[])
            n230 = Unbundle By Name(w620) -> ("Rename"=w621:T4[], "Delete"=w606:T4[])
            n231 = Unbundle By Name(w610) -> ("Rename"=w614:T4[], "Delete"=w597:T4[])
            n232 = Unbundle By Name(w584) -> ("Rename"=w586:T4[], "Delete"=w587:T4[])
            n233 = call "CRYSelect Changed Name.vi"("Option"=w593, "Inserted Name"=w622, "Origin Name"=w623, "Type"=w624) -> ("Wave"=w598:T3, "Result"=w583:T3, "Value"=w603:T3, "Cuve"=w608:T3)  [unwired: 4 in]
            n234 = Unbundle By Name(w598) -> ("Rename"=w595:T4[], "Delete"=w594:T4[])
            n235 = Unbundle By Name(w583) -> ("Rename"=w589:T4[], "Delete"=w590:T4[])
            n236 = Unbundle By Name(w603) -> ("Rename"=w602:T4[], "Delete"=w601:T4[])
            n237 = Insert Into Array(array=w600, new element=w601) -> (w599:T4[])  [unwired: 1 in]
            n238 = Insert Into Array(array=w616, new element=w602) -> (w617:T4[])  [unwired: 1 in]
            n239 = Insert Into Array(array=w614, new element=w595) -> (w615:T4[])  [unwired: 1 in]
            n240 = Insert Into Array(array=w597, new element=w594) -> (w596:T4[])  [unwired: 1 in]
            n241 = Insert Into Array(array=w586, new element=w589) -> (w585:T4[])  [unwired: 1 in]
            n242 = Insert Into Array(array=w587, new element=w590) -> (w588:T4[])  [unwired: 1 in]
            n243 = Unbundle By Name(w608) -> ("Rename"=w607:T4[], "Delete"=w605:T4[])
            n244 = Insert Into Array(array=w621, new element=w607) -> (w619:T4[])  [unwired: 1 in]
            n245 = Insert Into Array(array=w606, new element=w605) -> (w604:T4[])  [unwired: 1 in]
            n246 = Bundle By Name(cluster=w611, "Rename"=w617, "Delete"=w599) -> (w613:T3)
            n247 = Bundle By Name(cluster=w620, "Rename"=w619, "Delete"=w604) -> (w618:T3)
            n248 = Bundle By Name(cluster=w610, "Rename"=w615, "Delete"=w596) -> (w612:T3)
            n249 = Bundle By Name(cluster=w584, "Rename"=w585, "Delete"=w588) -> (w582:T3)
          }
        }
      }
      frame "Statistics" {
        n250 = call "CRYUnflatten Statistic.vi"("Flatten Statistics"=w738) -> ("Statistics"=w736:T26)  [unwired: 8 in, 2 out]
        n251 = Unbundle By Name(w736) -> ("Mode"=w717:u16, "Curves"=w734:string[], "Results"=w732:string[])
        n252 = case shown="1, 2" w717 {
          tunnel: [w741 w743] -> w733
          tunnel: w732 -> [w741 w747]
          tunnel: w713 -> [_ w746]
          tunnel: [bool[] [] w745] -> w730
          tunnel: [string[] [] w742] -> w718
          frame Default {
          }
          frame 1, 2 {
            n253 = for {
              tunnel: w747 -> [w756] mode=indexing
              tunnel: w746 -> [w755]
              tunnel: [w754] -> w745 mode=indexing
              shift-right: [w751] -> w743
              shift-left: string[] [] -> [w750]
              tunnel: [w748] -> w742 mode=indexing
              n254 = call "CRYSelect New Name.vi"("Result"=w755, "Type"="Statistics", "Option"="Result" ("Type"), "Name In"=w756) -> ("Change"=w754:bool, "Status"=w749:string, "Name Out"=w752:string)  [unwired: 5 in]
              n255 = case shown="\"Rename\"" w749 {
                selector: w749 -> [w759 w761 w767]
                tunnel: w750 -> [w758 w763 w766]
                tunnel: [w758 w762 w765] -> w751
                tunnel: [w759 w761 w767] -> w748
                tunnel: w752 -> [_ w760 w764]
                frame "Delete" {
                }
                frame "Rename" {
                  n256 = Insert Into Array(array=w763, new element=w760) -> (w762:string[])  [unwired: 1 in]
                }
                frame "Origin", Default {
                  n257 = Insert Into Array(array=w766, new element=w764) -> (w765:string[])  [unwired: 1 in]
                }
              }
            }
          }
        }
        n258 = case shown="0, 2" w717 {
          tunnel: [w770 w772] -> w735
          tunnel: w734 -> [w770 w777]
          tunnel: w728 -> [_ w776]
          tunnel: w727 -> [_ w775]
          tunnel: [bool[] [] w774] -> w731
          tunnel: [string[] [] w771] -> w719
          frame Default {
          }
          frame 0, 2 {
            n259 = for {
              tunnel: w777 -> [w785] mode=indexing
              tunnel: w776 -> [w787]
              tunnel: w775 -> [w786]
              tunnel: [w784] -> w774 mode=indexing
              shift-right: [w781] -> w772
              shift-left: string[] [] -> [w779]
              tunnel: [w778] -> w771 mode=indexing
              n260 = call "CRYSelect New Name.vi"("Type"="Statistics", "Option"="CurveValue" ("Type"), "Value"=w786, "Curve"=w787, "Name In"=w785) -> ("Change"=w784:bool, "Status"=w782:string, "Name Out"=w780:string)  [unwired: 4 in]
              n261 = case shown="\"Delete\"" w782 {
                selector: w782 -> [w790 w792 w798]
                tunnel: w779 -> [w789 w794 w796]
                tunnel: [w789 w793 w795] -> w781
                tunnel: [w790 w792 w798] -> w778
                tunnel: w780 -> [_ w791 w797]
                frame "Delete" {
                }
                frame "Rename" {
                  n262 = Insert Into Array(array=w794, new element=w791) -> (w793:string[])  [unwired: 1 in]
                }
                frame "Origin", Default {
                  n263 = Insert Into Array(array=w796, new element=w797) -> (w795:string[])  [unwired: 1 in]
                }
              }
            }
          }
        }
        n264 = Bundle By Name(cluster="Ref Data Statistics", "CurveValue"=w719, "Result"=w718) -> (w716:T1)
        n265 = Flatten To String(anything=w716) -> (data string=w715:string)  [unwired: 3 in, 2 out]
        n266 = Bundle By Name(cluster=w736, "Curves"=w735, "Results"=w733) -> (w729:T26)
        n267 = Or Array Elements(Boolean array=w731) -> (logical OR=w722:bool)
        n268 = Or Array Elements(Boolean array=w730) -> (logical OR=w721:bool)
        n269 = Compound Arithmetic op=OR(w722, w721) -> (w711:bool)
        n270 = call "CRYFlatten Statistic.vi"("Statistics"=w729) -> ("Flatten Statistics String"=w724:string)  [unwired: 10 in]
        n271 = Compound Arithmetic op=OR(w709, w711) -> (w710:bool)
        n272 = case shown="True" w710 {
          tunnel: w737 -> [_ w825]
          tunnel: w712 -> [_ w826]
          tunnel: w724 -> [_ w803]
          tunnel: w728 -> [w800 w817]
          tunnel: w727 -> [w799 w816]
          tunnel: [w800 w815] -> w726
          tunnel: [w799 w814] -> w725
          tunnel: w715 -> [_ w802]
          tunnel: w714 -> [_ w801]
          frame False {
          }
          frame True {
            n273 = flat-sequence {
              tunnel: [w835] -> w829
              tunnel: [w830] -> w828
              tunnel: w826 -> [w834]
              tunnel: [w832] -> w827
              tunnel: w803 -> [w830]
              tunnel: w829 -> [w840]
              tunnel: w828 -> [w837]
              tunnel: w827 -> [w841]
              tunnel: [w841] -> w824
              tunnel: [w840] -> w823
              tunnel: w825 -> [w839]
              tunnel: [w836] -> w822
              frame #0 {
                n274 = Build Array(w834) -> (w833:i32[])
                n275 = call "CRYGet Curve Library Data Name.vi"("nData"=w833, "sAction"="GetNamebyStep" ("sOption")) -> ("sNames"=w835:string[], "Type Out"=w832:string[])  [unwired: 6 in, 2 out]
              }
              frame #1 {
                n276 = call "CRYReplace Statistics Curve Name.vi"("Step Set up In"=w837, "Setup in"=w839, "Type In"="Apply") -> ("Inserted Names Out"=w836:string[])  [unwired: 7 in, 1 out]
              }
            }
            n277 = Unbundle By Name(w816) -> ("Rename"=w821:T4[], "Delete"=w805:T4[])
            n278 = Unbundle By Name(w817) -> ("Rename"=w818:T4[], "Delete"=w810:T4[])
            n279 = call "CRYSelect Changed Name.vi"("Option"=w801, "Ref Data"=w802, "Inserted Name"=w822, "Origin Name"=w823, "Type"=w824) -> ("Value"=w808:T3, "Cuve"=w813:T3)  [unwired: 3 in, 2 out]
            n280 = Unbundle By Name(w808) -> ("Rename"=w807:T4[], "Delete"=w806:T4[])
            n281 = Insert Into Array(array=w821, new element=w807) -> (w820:T4[])  [unwired: 1 in]
            n282 = Insert Into Array(array=w805, new element=w806) -> (w804:T4[])  [unwired: 1 in]
            n283 = Unbundle By Name(w813) -> ("Rename"=w812:T4[], "Delete"=w811:T4[])
            n284 = Insert Into Array(array=w810, new element=w811) -> (w809:T4[])  [unwired: 1 in]
            n285 = Insert Into Array(array=w818, new element=w812) -> (w819:T4[])  [unwired: 1 in]
            n286 = Bundle By Name(cluster=w816, "Rename"=w820, "Delete"=w804) -> (w814:T3)
            n287 = Bundle By Name(cluster=w817, "Rename"=w819, "Delete"=w809) -> (w815:T3)
          }
        }
      }
      frame "Auto Save" {
        n288 = call "CRYUnflatten Auto Save.vi"("Flatten Auto Save"=w856) -> ("Auto save"=w855:T27)  [unwired: 8 in, 2 out]
        n289 = Unbundle By Name(w855) -> ("save"=w854:enum16{"Data", "Results", "Waveforms"}, "Item Names"=w851:string[])
        n290 = case shown="\"Waveforms\"" w854 {
          tunnel: [w862 w874 w886] -> w850
          tunnel: w847 -> [w861 w873 w885]
          tunnel: w851 -> [w860 w872 w884]
          tunnel: w849 -> [w859 w871 w883]
          tunnel: w848 -> [w858 w870 w882]
          tunnel: w846 -> [_ _ w881]
          tunnel: [w857 w869 w880] -> w845
          frame "Data", Default {
            n291 = for {
              tunnel: [w867] -> w862 mode=indexing
              tunnel: w861 -> [_]
              tunnel: w860 -> [w866] mode=indexing
              tunnel: w859 -> [w865]
              tunnel: w858 -> [w864]
              tunnel: [w863] -> w857 mode=indexing
              n292 = call "CRYSelect New Name.vi"("Type"="Auto Save", "Value"=w864, "Curve"=w865, "Name In"=w866) -> ("Change"=w863:bool, "Name Out"=w867:string)  [unwired: 5 in, 1 out]
            }
          }
          frame "Results" {
            n293 = for {
              tunnel: [w878] -> w874 mode=indexing
              tunnel: w873 -> [w876]
              tunnel: w872 -> [w877] mode=indexing
              tunnel: w871 -> [_]
              tunnel: w870 -> [_]
              tunnel: [w875] -> w869 mode=indexing
              n294 = call "CRYSelect New Name.vi"("Result"=w876, "Type"="Results", "Name In"=w877) -> ("Change"=w875:bool, "Name Out"=w878:string)  [unwired: 6 in, 1 out]
            }
          }
          frame "Waveforms" {
            n295 = for {
              tunnel: [w890] -> w886 mode=indexing
              tunnel: w885 -> [_]
              tunnel: w884 -> [w889] mode=indexing
              tunnel: w883 -> [_]
              tunnel: w882 -> [_]
              tunnel: w881 -> [w888]
              tunnel: [w887] -> w880 mode=indexing
              n296 = call "CRYSelect New Name.vi"("Type"="Wave", "Wave"=w888, "Name In"=w889) -> ("Change"=w887:bool, "Name Out"=w890:string)  [unwired: 6 in, 1 out]
            }
          }
        }
        n297 = Bundle By Name(cluster=w855, "Item Names"=w850) -> (w852:T27)
        n298 = Or Array Elements(Boolean array=w845) -> (logical OR=w844:bool)
        n299 = call "CRYFlatten Auto Save.vi"("Auto Save"=w852) -> ("Auto Save flattened"=w853:string)  [unwired: 10 in]
      }
    }
    n300 = Compound Arithmetic op=OR(w19, w21) -> (w20:bool)
    n301 = case shown="True" w20 {
      tunnel: w43 -> [_ w48]
      tunnel: w23 -> [_ w46]
      frame False {
      }
      frame True {
        n302 = call "CRYStep Update.vi"("sOption"="ChangeName", "Seq-step setup"=w48, "Proper VI No"=w46) -> ()  [unwired: 9 in]
      }
    }
  }
